vi "S3_Send API Request v4.vi"(6 "request body":string, 7 "Authorization":string, 8 "error in (no error)":errorcluster, 9 "HTTP-Verb":string, 10 "Host String":string, 11 "Client Handle In":T2) -> (0 "error out":errorcluster, 1 "Call Result":T1, 2 "response body":string, 3 "response headers":string, 4 "Redirect endpoint":string)   [LabVIEW 2015, in "LV Interface for Amazon S3.lvlib"]
uses:
  LV Interface for Amazon S3.lvlib
  <vilib>/httpClient/ClientHandle.ctl
  Typedefs/AMZ_S3_Call Results.ctl
  <vilib>/httpClient/PUTBuffer.vi
  <vilib>/httpClient/POSTBuffer.vi
  <vilib>/httpClient/LabVIEWHTTPClient.lvlib
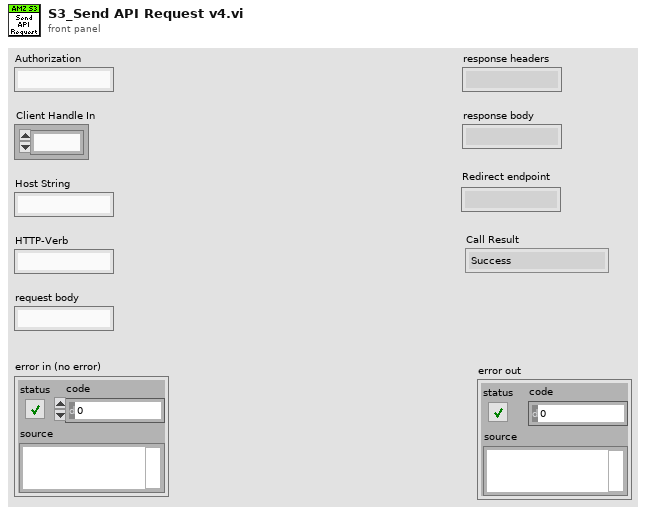
[diagram p1: front panel]
types:
  T1 = typedef "LV Interface for Amazon S3.lvlib/AMZ_S3_Call Results.ctl" = enum16{"Success", "UndefinedError", "AccessDenied", "AccountProblem", "AmbiguousGrantByEmailAddress", "BadDigest", "BucketAlreadyExists", "BucketAlreadyOwnedByYou", "BucketNotEmpty", "CredentialsNotSupported", "CrossLocationLoggingProhibited", "EntityTooSmall", "EntityTooLarge", "ExpiredToken", "IllegalVersioningConfigurationException", "IncompleteBody", "IncorrectNumberOfFilesInPostRequest", "InlineDataTooLarge", "InternalError", "InvalidAccessKeyId", "InvalidAddressingHeader", "InvalidArgument", "InvalidBucketName", "InvalidDigest", "InvalidLocationConstraint", "InvalidPart", "InvalidPartOrder", "InvalidPayer", "InvalidPolicyDocument", "InvalidRange", "InvalidSecurity", "InvalidSOAPRequest", "InvalidStorageClass", "InvalidTargetBucketForLogging", "InvalidToken", "InvalidURI", "KeyTooLong", "MalformedACLError", "MalformedPOSTRequest", "MalformedXML", "MaxMessageLengthExceeded", "MaxPostPreDataLengthExceededError", "MetadataTooLarge", "MethodNotAllowed", "MissingAttachment", "MissingContentLength", "MissingRequestBodyError", "MissingSecurityElement", "MissingSecurityHeader", "NoLoggingStatusForKey", "NoSuchBucket", "NoSuchKey", "NoSuchUpload", "NoSuchVersion", "NotImplemented", "NotSignedUp", "OperationAborted", "PermanentRedirect", "PreconditionFailed", "Redirect", "RequestIsNotMultiPartContent", "RequestTimeout", "RequestTimeTooSkewed", "RequestTorrentOfBucketError", "SignatureDoesNotMatch", "SlowDown", "TemporaryRedirect", "TokenRefreshRequired", "TooManyBuckets", "UnexpectedContent", "UnresolvableGrantByEmailAddress", "UserKeyMustBeSpecified", "LabVIEWError"}
  T2 = typedef "LabVIEWHTTPClient.lvlib/ClientHandle.ctl" = refnum<k1>
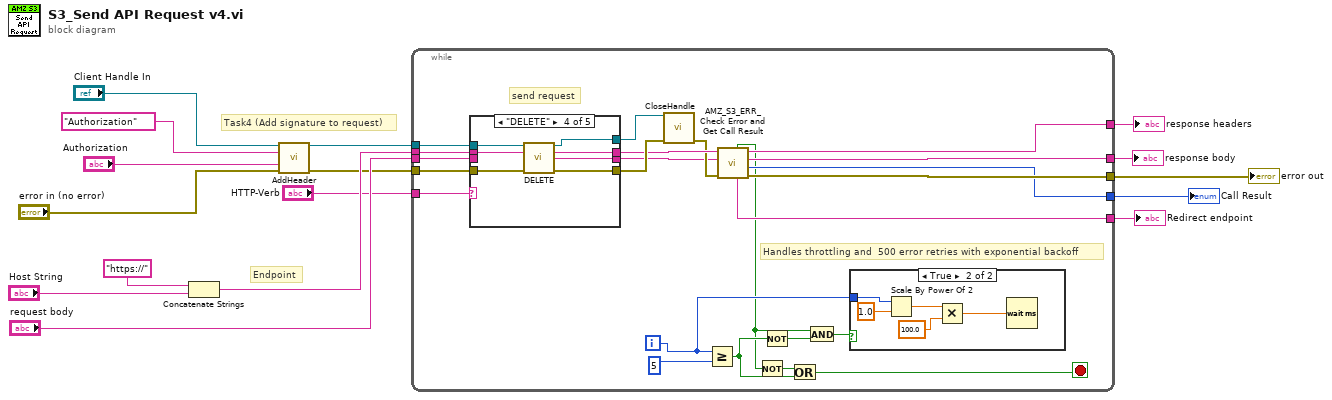
[diagram p0: block diagram]
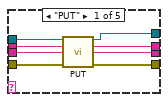
[diagram p3: hidden frame]
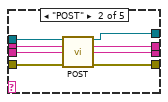
[diagram p4: hidden frame]
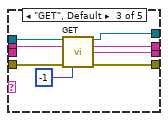
[diagram p5: hidden frame]
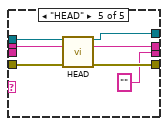
[diagram p6: hidden frame]
diagram:
  # "Endpoint"
  # "Task4 (Add signature to request)"
  n1 = Concatenate Strings("https://" ("string"), "Host String") -> (w15:string)
  n2 = call <vilib>:"AddHeader.vi"("client handle"="Client Handle In", "header"="Authorization", "value"="Authorization", "error in (no error)"="error in (no error)") -> ("client handle out"=w9:T2, "error out"=w12:errorcluster)  [unwired: 10 in]
  n3 = while {
    tunnel: w9 -> [w36]
    tunnel: [w18] -> w1
    tunnel: w15 -> [w38]
    tunnel: [w30] -> w4
    tunnel: "request body" -> [w39]
    tunnel: [w29] -> w3
    tunnel: "HTTP-Verb" -> [w35]
    tunnel: [w20] -> w2
    tunnel: w12 -> [w37]
    tunnel: [w31] -> w5
    i -> [w25]
    stop <- w24 stop-if-true
    # "Handles throttling and  500 error retries with exponential backoff"
    # "send request"
    n4 = case shown="\"DELETE\"" w35 {
      tunnel: [w47 w60 w67 w70 "" ("body")] -> w19
      tunnel: [w46 w59 w68 w69 w82] -> w32
      tunnel: w38 -> [w51 w58 w64 w73 w80]
      tunnel: w36 -> [w52 w57 w63 w72 w78]
      tunnel: w39 -> [w50 w56 _ _ _]
      tunnel: w37 -> [w49 w55 w65 w74 w79]
      tunnel: [w48 w54 w66 w75 w81] -> w33
      tunnel: [w45 w53 w62 w71 w77] -> w34
      frame "PUT" {
        n5 = call-poly <vilib>:"PUT.vi"("client handle"=w52, "url"=w51, "buffer"=w50, "error in (no error)"=w49) -> ("client handle out"=w45:T2, "headers"=w46:string, "body"=w47:string, "error out"=w48:errorcluster)  [unwired: 8 in]
      }
      frame "POST" {
        n6 = call-poly <vilib>:"POST.vi"("client handle"=w57, "url"=w58, "buffer"=w56, "error in (no error)"=w55) -> ("client handle out"=w53:T2, "headers"=w59:string, "body"=w60:string, "error out"=w54:errorcluster)  [unwired: 8 in]
      }
      frame "GET", Default {
        n7 = call <vilib>:"GET.vi"("client handle"=w63, "url"=w64, "error in (no error)"=w65, "timeout (10000)"=-1) -> ("client handle out"=w62:T2, "headers"=w68:string, "body"=w67:string, "error out"=w66:errorcluster)  [unwired: 8 in]
      }
      frame "DELETE" {
        n8 = call <vilib>:"DELETE.vi"("client handle"=w72, "url"=w73, "error in (no error)"=w74) -> ("client handle out"=w71:T2, "headers"=w69:string, "body"=w70:string, "error out"=w75:errorcluster)  [unwired: 9 in]
      }
      frame "HEAD" {
        n9 = call <vilib>:"HEAD.vi"("client handle"=w78, "url"=w80, "error in (no error)"=w79) -> ("client handle out"=w77:T2, "headers"=w82:string, "error out"=w81:errorcluster)  [unwired: 10 in]
      }
    }
    n10 = call <vilib>:"CloseHandle.vi"("client handle"=w34, "error in (no error)"=w33) -> ("error out"=w28:errorcluster)  [unwired: 13 in]
    n11 = Greater Or Equal?(x=w25, y=5) -> (x >= y?=w21:bool)
    n12 = call "AMZ_S3_ERR_Check Error and Get Call Result.vi"("error in (no error)"=w28, "Response body"=w19, "Response header"=w32) -> ("error out"=w31:errorcluster, "Call Result"=w18:T1, "Response body dup"=w29:string, "Response header dup"=w30:string, "Redirect endpoint"=w20:string, "500 Or Throttled?"=w17:bool)  [unwired: 3 in]
    n13 = Not(x=w17) -> (.not. x?=w27:bool)
    n14 = Not(x=w21) -> (.not. x?=w22:bool)
    n15 = Or(x=w27, y=w21) -> (x .or. y?=w24:bool)
    n16 = And(x=w17, y=w22) -> (x .and. y?=w23:bool)
    n17 = case shown="True" w23 {
      tunnel: w25 -> [_ w43]
      frame False {
        # "Do not reattempt call"
      }
      frame True {
        n18 = Scale By Power Of 2(n=w43, x=1.0) -> (x*2^n=w41:dbl)
        n19 = Multiply(x=w41, y=100.0) -> (x*y=w42:dbl)
        n20 = Wait (ms)(milliseconds to wait=w42) -> ()  [unwired: 1 out]
      }
    }
  }
  "response headers" <- w4
  "response body" <- w3
  "error out" <- w5
  "Redirect endpoint" <- w2
  "Call Result" <- w1
